vi "Build Single Tone Results.vi"(6 "Channel name":string, 7 "FFT":cluster{"x0":dbl, "dx":dbl, "magnitude":dbl[]}, 9 "Time domain":waveform(dbl), 10 "Single tone results":T2, 11 "Meas Results In":T1 {"ENOB" format="%_6g"; "THD (dB)" format="%_6g"; "SINAD (dB)" format="%_6g"; "SNR (dB)" format="%_6g"; "SFDR (dBc)" format="%_6g"; "Amplitude (dB)" format="%_6g"; "Amplitude (V)" format="%_6g"; "Frequency (Hz)" format="%_6g"; "df" format="%_6g"; "f0" format="%_6g"; "dt" format="%_6g"; "Frequency domain" format="%_6g"; "Time domain" format="%_6g"}) -> (3 "Meas Results Out":T1 {"ENOB" format="%_6g"; "THD (dB)" format="%_6g"; "SINAD (dB)" format="%_6g"; "SNR (dB)" format="%_6g"; "SFDR (dBc)" format="%_6g"; "Amplitude (dB)" format="%_6g"; "Amplitude (V)" format="%_6g"; "Frequency (Hz)" format="%_6g"; "df" format="%_6g"; "f0" format="%_6g"; "dt" format="%_6g"; "Frequency domain" format="%_6g"; "Time domain" format="%_6g"})   [LabVIEW 2021, in "Single Tone_DAC.lvlib"]
uses:
  Measurement Results.ctl
  Single Tone_DAC.lvlib
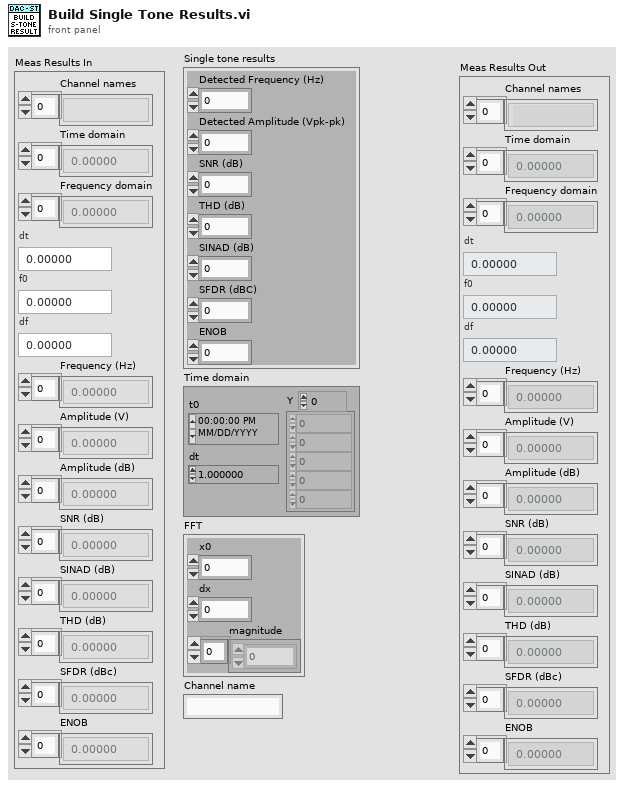
[diagram p1: front panel]
types:
  T1 = typedef "Single Tone_DAC.lvlib/Measurement Results.ctl" = cluster{"Channel names":string[], "Time domain":dbl[], "Frequency domain":dbl[], "dt":dbl, "f0":dbl, "df":dbl, "Frequency (Hz)":dbl[], "Amplitude (V)":dbl[], "Amplitude (dB)":dbl[], "SNR (dB)":dbl[], "SINAD (dB)":dbl[], "THD (dB)":dbl[], "SFDR (dBc)":dbl[], "ENOB":dbl[]}
  T2 = cluster{"Detected Frequency (Hz)":dbl, "Detected Amplitude (Vpk-pk)":dbl, "SNR (dB)":dbl, "THD (dB)":dbl, "SINAD (dB)":dbl, "SFDR (dBC)":dbl, "ENOB":dbl}
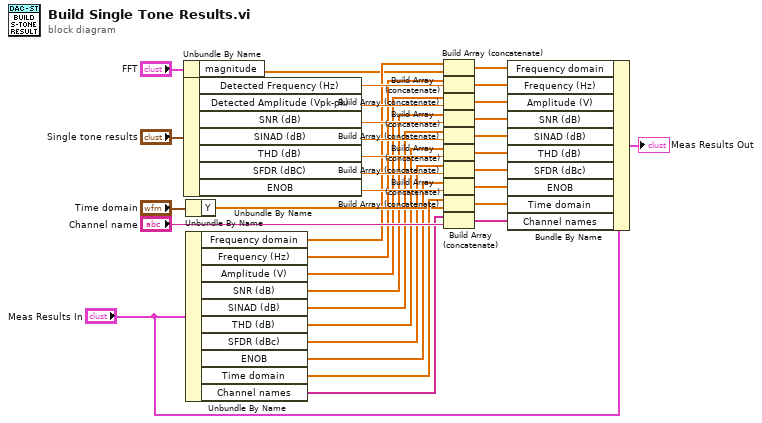
[diagram p0: block diagram]
diagram:
  n1 = Unbundle By Name("FFT") -> ("magnitude"=w4:dbl[])
  n2 = Unbundle By Name("Single tone results") -> ("Detected Frequency (Hz)"=w23:dbl, "Detected Amplitude (Vpk-pk)"=w25:dbl, "SNR (dB)"=w27:dbl, "SINAD (dB)"=w29:dbl, "THD (dB)"=w31:dbl, "SFDR (dBC)"=w33:dbl, "ENOB"=w21:dbl)
  n3 = Unbundle By Name("Time domain") -> ("Y"=w14:dbl[])
  n4 = Unbundle By Name("Meas Results In") -> ("Frequency domain"=w5:dbl[], "Frequency (Hz)"=w6:dbl[], "Amplitude (V)"=w7:dbl[], "SNR (dB)"=w8:dbl[], "SINAD (dB)"=w9:dbl[], "THD (dB)"=w10:dbl[], "SFDR (dBc)"=w11:dbl[], "ENOB"=w12:dbl[], "Time domain"=w15:dbl[], "Channel names"=w16:string[])
  n5 = Build Array (concatenate)(w5, w4) -> (w3:dbl[])
  n6 = Build Array (concatenate)(w6, w23) -> (w24:dbl[])
  n7 = Build Array (concatenate)(w7, w25) -> (w26:dbl[])
  n8 = Build Array (concatenate)(w8, w27) -> (w28:dbl[])
  n9 = Build Array (concatenate)(w9, w29) -> (w30:dbl[])
  n10 = Build Array (concatenate)(w10, w31) -> (w32:dbl[])
  n11 = Build Array (concatenate)(w11, w33) -> (w34:dbl[])
  n12 = Build Array (concatenate)(w12, w21) -> (w22:dbl[])
  n13 = Build Array (concatenate)(w15, w14) -> (w13:dbl[])
  n14 = Build Array (concatenate)(w16, "Channel name") -> (w19:string[])
  n15 = Bundle By Name(cluster="Meas Results In", "Frequency domain"=w3, "Frequency (Hz)"=w24, "Amplitude (V)"=w26, "SNR (dB)"=w28, "SINAD (dB)"=w30, "THD (dB)"=w32, "SFDR (dBc)"=w34, "ENOB"=w22, "Time domain"=w13, "Channel names"=w19) -> (→"Meas Results Out":T1)
